vi "Read Port simulated.vi"(8 "error in (no error)":errorcluster, 10 "Port":dbl, 11 "Simulated Device in":refnum<class "Simulated Device.lvclass">) -> (0 "error out":errorcluster, 1 "Response":string, 2 "Binary Number":T1, 3 "Simulated Device out":refnum<class "Simulated Device.lvclass">)   [LabVIEW 2020, in "Simulated Device.lvclass"]
uses:
  Simulated Device.lvclass
  c1c6cbbc-b879-4ed8-a3ee-69cc487a1d55.vi
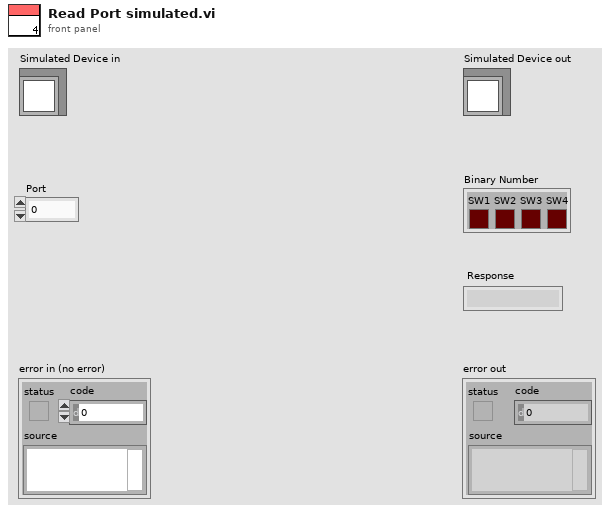
[diagram p1: front panel]
types:
  T1 = cluster{"SW1":bool, "SW2":bool, "SW3":bool, "SW4":bool, "[4]":bool, "[5]":bool, "[6]":bool, "[7]":bool, "[8]":bool}
  T2 = enum16{"Write", "Read", "Config", "Reset", "Close"}
  T3 = cluster{"[0]":bool, "[1]":bool, "[2]":bool, "[3]":bool, "[4]":bool, "[5]":bool, "[6]":bool, "[7]":bool, "[8]":bool}
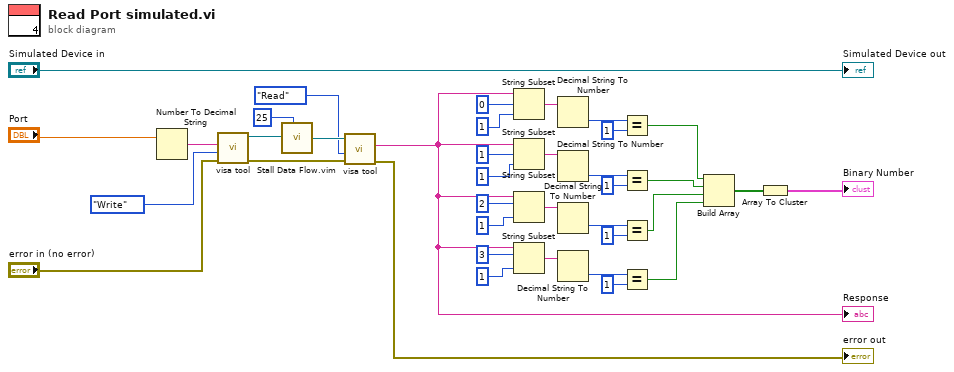
[diagram p0: block diagram]
diagram:
  n1 = Number To Decimal String(number="Port") -> (decimal integer string=w37:string)  [unwired: 1 in]
  n2 = call "visa tool.vi"("error in (no error)"="error in (no error)", "Opciones"=T2."Write", "Write"=w37) -> ("error out"=w31:errorcluster, "VISA com port 2"=w35:refnum<visa-resource-name>)  [unwired: 6 in, 1 out]
  n3 = call "Stall Data Flow.vim"("value in"=w35, "milliseconds to wait"=u32 25) -> ("value out"=w34:refnum<visa-resource-name>)  [unwired: 1 out]
  n4 = call "visa tool.vi"("error in (no error)"=w31, "Opciones"=T2."Read", "VISA com port"=w34) -> ("error out"=→"error out":errorcluster, "Read"=w4:string)  [unwired: 6 in, 1 out]
  "Response" <- w4
  n5 = String Subset(string=w4, offset (0)=0, length (rest)=1 ("length (rest)")) -> (substring=w22:string)
  n6 = String Subset(string=w4, offset (0)=1, length (rest)=1 ("length (rest)")) -> (substring=w21:string)
  n7 = String Subset(string=w4, offset (0)=2, length (rest)=1 ("length (rest)")) -> (substring=w20:string)
  n8 = String Subset(string=w4, offset (0)=3, length (rest)=1 ("length (rest)")) -> (substring=w19:string)
  n9 = Decimal String To Number(string=w22) -> (number=w18:i32)  [unwired: 2 in, 1 out]
  n10 = Decimal String To Number(string=w21) -> (number=w13:i32)  [unwired: 2 in, 1 out]
  n11 = Decimal String To Number(string=w20) -> (number=w12:i32)  [unwired: 2 in, 1 out]
  n12 = Decimal String To Number(string=w19) -> (number=w11:i32)  [unwired: 2 in, 1 out]
  n13 = Equal?(x=w18, y=1) -> (x = y?=w10:bool)
  n14 = Equal?(x=w13, y=1) -> (x = y?=w9:bool)
  n15 = Equal?(x=w12, y=1) -> (x = y?=w8:bool)
  n16 = Equal?(x=w11, y=1) -> (x = y?=w7:bool)
  n17 = Build Array(w10, w9, w8, w7) -> (w6:bool[])
  n18 = Array To Cluster(array=w6) -> (cluster=→"Binary Number":T3)
  "Simulated Device out" <- "Simulated Device in"
